vi "Pockels Cal-Force cal setup.vi"(8 "error in (no error)":errorcluster, 11 "Function":enum16{"Set", "Recover"}(ring)) -> (0 "error out":errorcluster)   [LabVIEW 2013]
uses:
  Global Variables/gl_UI Ctrl Refs.vi
  Globals/gl_Calibration globals.vi
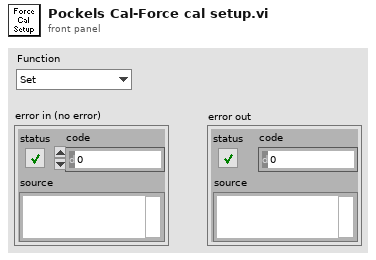
[diagram p1: front panel]
types:
  T1 = typedef "Laser control knob.ctl" = u16
  T2 = typedef "UI ctrl refs cluster.ctl" = cluster{"Top level VI path":path, "Top level VI ref":refnum<vi>, "User menu ref":refnum<k9>, "Sub Panel control":refnum<vi>, "Imaging Param Tab":refnum<vi>, "Occurrence-Start drivers":refnum<k4>, "Occurrence-Speed logging initialised":refnum<k4>, "Occurrence-XYZ stage initialised":refnum<k4>, "Exit button":refnum<vi>, "Status ind":refnum<vi>, "Return to Origin":refnum<vi>, "Speed Logging":refnum<vi>, "Time Lapse":refnum<vi>, "Live Imaging":refnum<vi>, "AOL Z Stack":refnum<vi>, "Motor Z Stack":refnum<vi>, "Funct Acq button":refnum<vi>, "Hard Shutter":refnum<vi>, "Virtual Shutter":refnum<vi>, "Laser Power":refnum<vi>, "AOL Mode":refnum<vi>, "Frame Size":refnum<vi>, "Field of View":refnum<vi>, "Dwell Time":refnum<vi>, "Zoom":refnum<vi>, "AOL Z":refnum<vi>, "Objective":refnum<vi>, "Axis":refnum<vi>, "Paths & Names":refnum<vi>, "Experiment folder path (ind.)":refnum<vi>, "Last State (Ind.)":refnum<vi>, "Laser wavelength ind (nm)":refnum<vi>, "Averages":refnum<vi>, "Angle (degrees)":refnum<vi>, "X centre":refnum<vi>, "Y centre":refnum<vi>, "Plane Mode":refnum<vi>, "# Planes":refnum<vi>, "Z Start":refnum<vi>, "Z Stop":refnum<vi>, "Z Step":refnum<vi>, "PMT 1":refnum<vi>, "PMT 2":refnum<vi>, "Stage XYZ Position":refnum<vi>, "Pockels@Z Start":refnum<vi>, "Pockels@Z Stop":refnum<vi>, "Obtain Z Start":refnum<vi>, "Obtain Z Stop":refnum<vi>, "Live stim.trig.period":refnum<vi>, "Live stim.trig.enable":refnum<vi>, "Funct. Acq. Pockels Modulation":refnum<vi>, "Enable Video Recording":refnum<vi>, "Video Record-Live Imaging":refnum<vi>, "Video Record-Funct acq":refnum<vi>, "AOL Z-stack Chirps Ready (ind)":refnum<vi>, "Center freq ind (nm)":refnum<vi>, "Logging queue (ind)":refnum<vi>, "Back aperture power (ind.)":refnum<vi>, "Power after objective (ind.)":refnum<vi>, "Switch user":refnum<vi>}
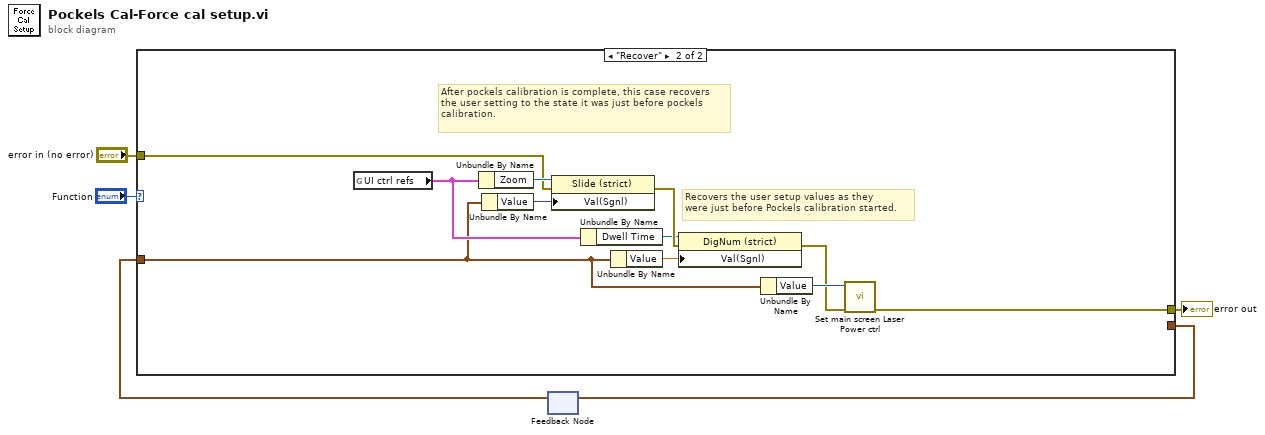
[diagram p0: block diagram]
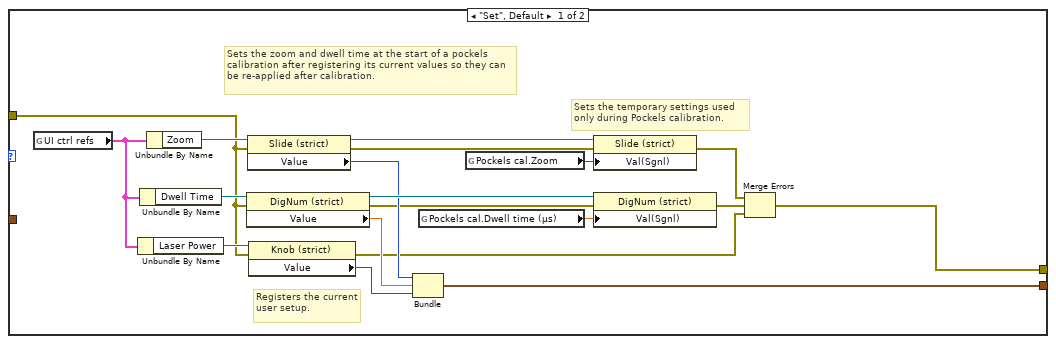
[diagram p2: hidden frame]
diagram:
  n1 = feedback #1() -> (w1:cluster{"Value":i8, "Value":dbl, "Value":T1})  [unwired: 1 in]
  n2 = case shown="\"Recover\"" "Function" {
    tunnel: [w8 w25] -> w5
    tunnel: "error in (no error)" -> [w6 w33]
    tunnel: [w22 _] -> w2
    tunnel: w1 -> [_ w28]
    frame "Set", Default {
      # "Registers the current user setup."
      # "Sets the temporary settings used \nonly during Pockels calibration."
      # "Sets the zoom and dwell time at the start of a pockels calibration after registering its current values so they can be re-applied after calibration."
      n3 = global read "gl_UI Ctrl Refs.vi" "UI ctrl refs"() -> (w14:T2)
      n4 = Unbundle By Name(w14) -> ("Laser Power"=w15:refnum<vi>)
      n5 = Unbundle By Name(w14) -> ("Dwell Time"=w19:refnum<vi>)
      n6 = Unbundle By Name(w14) -> ("Zoom"=w21:refnum<vi>)
      n7 = property class="DigNum (strict)"(reference=w19, error in=w6) -> (reference out=w18:refnum<vi>, error out=w11:errorcluster, "Value"=w16:dbl)
      n8 = property class="Slide (strict)"(reference=w21, error in=w6) -> (reference out=w20:refnum<vi>, error out=w12:errorcluster, "Value"=w17:i8)
      n9 = property class="Knob (strict)"(reference=w15, error in=w6) -> (error out=w7:errorcluster, "Value"=w13:T1)  [unwired: 1 out]
      n10 = Bundle("Value"=w17, "Value"=w16, "Value"=w13) -> (w22:cluster{"Value":i8, "Value":dbl, "Value":T1})  [unwired: 1 in]
      n11 = global read "gl_Calibration globals.vi" "Pockels cal.Dwell time (µs)"() -> (w24:dbl)
      n12 = global read "gl_Calibration globals.vi" "Pockels cal.Zoom"() -> (w23:u8)
      n13 = property class="Slide (strict)"(reference=w20, error in=w12, "Val(Sgnl)"=w23) -> (error out=w10:errorcluster)  [unwired: 1 out]
      n14 = property class="DigNum (strict)"(reference=w18, error in=w11, "Val(Sgnl)"=w24) -> (error out=w9:errorcluster)  [unwired: 1 out]
      n15 = Merge Errors(w10, w9, w7) -> (w8:errorcluster)
    }
    frame "Recover" {
      # "Recovers the user setup values as they \nwere just before Pockels calibration started."
      # "After pockels calibration is complete, this case recovers the user setting to the state it was just before pockels calibration."
      n16 = global read "gl_UI Ctrl Refs.vi" "UI ctrl refs"() -> (w29:T2)
      n17 = Unbundle By Name(w29) -> ("Zoom"=w35:refnum<vi>)
      n18 = Unbundle By Name(w28) -> ("Value"=w31:i8)
      n19 = property class="Slide (strict)"(reference=w35, error in=w33, "Val(Sgnl)"=w31) -> (error out=w34:errorcluster)  [unwired: 1 out]
      n20 = Unbundle By Name(w29) -> ("Dwell Time"=w32:refnum<vi>)
      n21 = Unbundle By Name(w28) -> ("Value"=w30:dbl)
      n22 = property class="DigNum (strict)"(reference=w32, error in=w34, "Val(Sgnl)"=w30) -> (error out=w26:errorcluster)  [unwired: 1 out]
      n23 = Unbundle By Name(w28) -> ("Value"=w27:T1)
      n24 = call "Set main screen Laser Power ctrl.vi"("error in (no error)"=w26, "Value (Signaling)"=w27) -> ("error out"=w25:errorcluster)  [unwired: 9 in]
    }
  }
  "error out" <- w5
  n25 = feedback-in #1(w2) -> ()
